vi "CloseTApe.vi"(8 "error in (no error)":errorcluster, 11 "VISA Refnum in":refnum<visa-resource-name>) -> (0 "error out":errorcluster)   [LabVIEW 2011]
uses:
  <instrlib>/Newport ESP301/Newport ESP301.lvlib
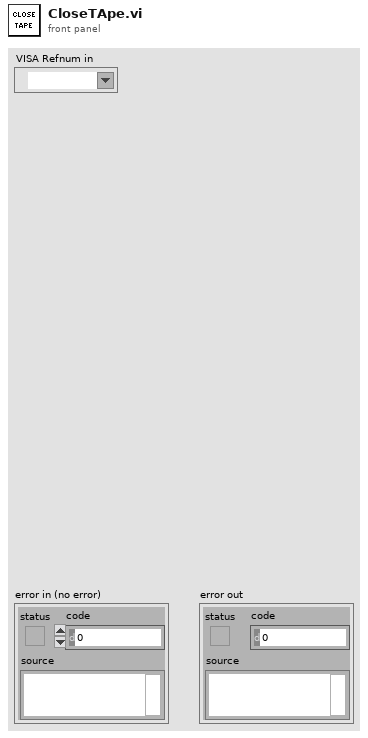
[diagram p1: front panel]
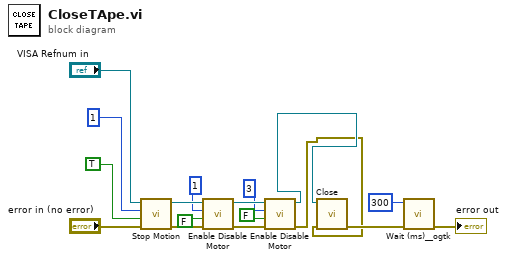
[diagram p0: block diagram]
diagram:
  n1 = call <instrlib>:"Stop Motion.vi"("error in (no error)"="error in (no error)", "Stop all axes (F)"=TRUE, "Axis (1)"=1, "VISA resource name"="VISA Refnum in") -> ("error out"=w5:errorcluster, "VISA resource name out"=w10:refnum<visa-resource-name>)  [unwired: 2 in]
  n2 = call <instrlib>:"Enable Disable Motor.vi"("error in (no error)"=w5, "Action (OFF)"=FALSE, "Axis (1)"=1, "VISA resource name"=w10) -> ("error out"=w4:errorcluster, "VISA resource name out"=w7:refnum<visa-resource-name>)  [unwired: 2 in]
  n3 = call <instrlib>:"Enable Disable Motor.vi"("error in (no error)"=w4, "Action (OFF)"=FALSE, "Axis (1)"=3, "VISA resource name"=w7) -> ("error out"=w1:errorcluster, "VISA resource name out"=w2:refnum<visa-resource-name>)  [unwired: 2 in]
  n4 = call <instrlib>:"Close.vi"("error in (no error)"=w1, "VISA resource name"=w2) -> ("error out"=w14:errorcluster)  [unwired: 9 in]
  n5 = call <userlib>:"Wait (ms)__ogtk.vi"("error in (no error)"=w14, "milliseconds to wait"=u32 300) -> ("error out"=→"error out":errorcluster)  [unwired: 8 in, 1 out]
